vi "Add Collision Component .vi"(11 "Game Board in":refnum<class "Game Board.lvclass">) -> (3 "Game Board out":refnum<class "Game Board.lvclass">)   [LabVIEW 2024, in "Game Board.lvclass"]
doc: "MIT Licence\nCopyright (c) 2024 David Grollier"
uses:
  Game Board.lvclass
  Game Board.lvclass/Game Board.ctl
  Collision/Collision.lvclass
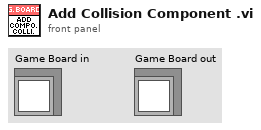
[diagram p1: front panel]
types:
  T1 = map{string, refnum<class "Game Board Component.lvclass">}
  T2 = typedef "Game Board.lvclass/Combinations Collision.ctl" = cluster{"Collision":refnum<class "Collision.lvclass">, "Combination":string[]}
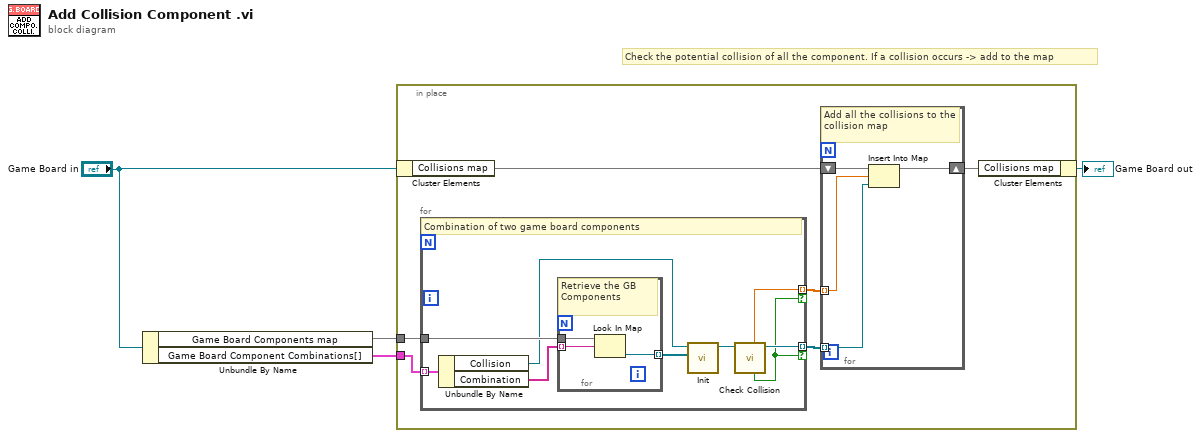
[diagram p0: block diagram]
diagram:
  # "Check the potential collision of all the component. If a collision occurs -> add to the map"
  n1 = Unbundle By Name("Game Board in") -> ("Game Board Components map"=w3:T1, "Game Board Component Combinations[]"=w2:T2[])
  n2 = in-place {
    in-place-border: w3 -> [w10]
    in-place-border: w2 -> [w9]
    n3 = in-place-cluster #1("Game Board in") -> ("Collisions map"=w8:map{dbl, refnum<class "Collision.lvclass">})
    n4 = for {
      tunnel: w9 -> [w23] mode=indexing
      tunnel: w10 -> [w21]
      tunnel: [w17] -> w7 mode=indexing if=w15
      tunnel: [w16] -> w6 mode=indexing if=w15
      # "Combination of two game board components"
      n5 = Unbundle By Name(w23) -> ("Collision"=w18:refnum<class "Collision.lvclass">, "Combination"=w22:string[])
      n6 = for {
        tunnel: w22 -> [w25] mode=indexing
        tunnel: w21 -> [w26]
        tunnel: [w24] -> w20 mode=indexing
        # "Retrieve the GB Components"
        n7 = Look In Map(map=w26, key=w25) -> (value=w24:refnum<class "Game Board Component.lvclass">)  [unwired: 1 in, 1 out]
      }
      n8 = call "Init.vi"("Game Board Components[2] in"=w20, "Collision in"=w18) -> ("Collision out"=w19:refnum<class "Collision.lvclass">)  [unwired: 9 in]
      n9 = call "Check Collision.vi"("Collision in"=w19) -> ("Collision out"=w17:refnum<class "Collision.lvclass">, "Collision?"=w15:bool, "Dichotomie factor out"=w16:dbl)  [unwired: 8 in]
    }
    n10 = for {
      shift-right: [w11] -> w5
      shift-left: w8 -> [w13]
      tunnel: w7 -> [w14] mode=indexing
      tunnel: w6 -> [w12] mode=indexing
      # "Add all the collisions to the collision map"
      n11 = Insert Into Map(map in=w13, key=w12, value=w14) -> (map out=w11:map{dbl, refnum<class "Collision.lvclass">})  [unwired: 2 out]
    }
    n12 = in-place-cluster #1("Collisions map"=w5) -> (→"Game Board out":refnum<class "Game Board.lvclass">)
  }
